vi "Configure Channel (mA Scale).vi"(0 "VISA resource name":refnum<visa-resource-name>, 1 "Scaling":T2={"Floating Point Position (2)"=2, "Lower Scaling (0.00)"=0.0, "Upper Scaling (100.00)"=100.0, "Unit Character (\"\")"=""} {"Upper Scaling (100.00)" format="%_6g"; "Lower Scaling (0.00)" format="%_6g"; "Floating Point Position (2)" min=0 max=5 step=1}, 5 "Channel (0001)":string="0001", 7 "Enable Channel (True)":bool=TRUE, 9 "Range And Span":T1={"mA Range (0 : 0-20mA)"=0, "Enable Span (False)"=FALSE, "Lower Span (0.000)"=0.0, "Upper Span (20.000)"=20.0, "Bias (0)"=0.0} {"mA Range (0 : 0-20mA)" items=["0-20mA"]; "Bias (0)" format="%_6g"; "Upper Span (20.000)" step=0.001 format="%.3g"; "Lower Span (0.000)" step=0.001 format="%.3g"}, 11 "error in (no error)":errorcluster) -> (4 "VISA resource name out":refnum<visa-resource-name>, 6 "Channel":string, 15 "error out":errorcluster)   [LabVIEW 2020, in "Yokogawa GX Series.lvlib"]
doc: "Sets the input range as voltage.\n\nCommand: SRangeAI"
uses:
  <instrlib>/Yokogawa GX Series/Yokogawa GX Series.lvlib
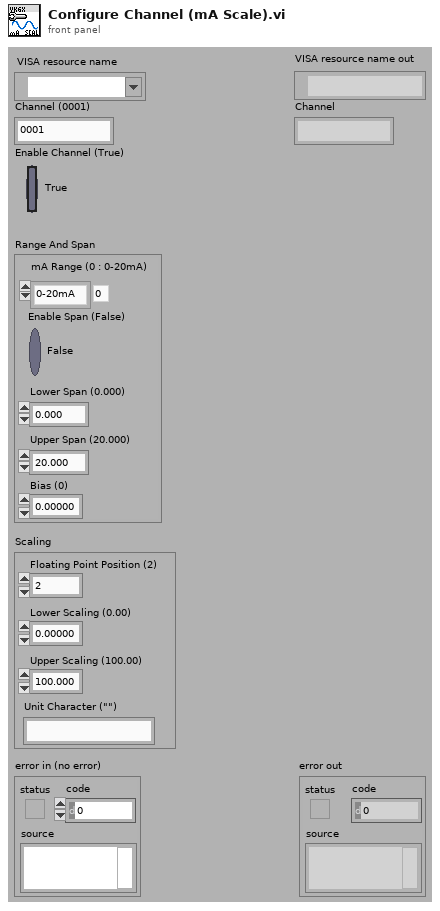
[diagram p1: front panel]
types:
  T1 = cluster{"mA Range (0 : 0-20mA)":i32, "Enable Span (False)":bool, "Lower Span (0.000)":dbl, "Upper Span (20.000)":dbl, "Bias (0)":dbl}
  T2 = cluster{"Floating Point Position (2)":i32, "Lower Scaling (0.00)":dbl, "Upper Scaling (100.00)":dbl, "Unit Character (\"\")":string}
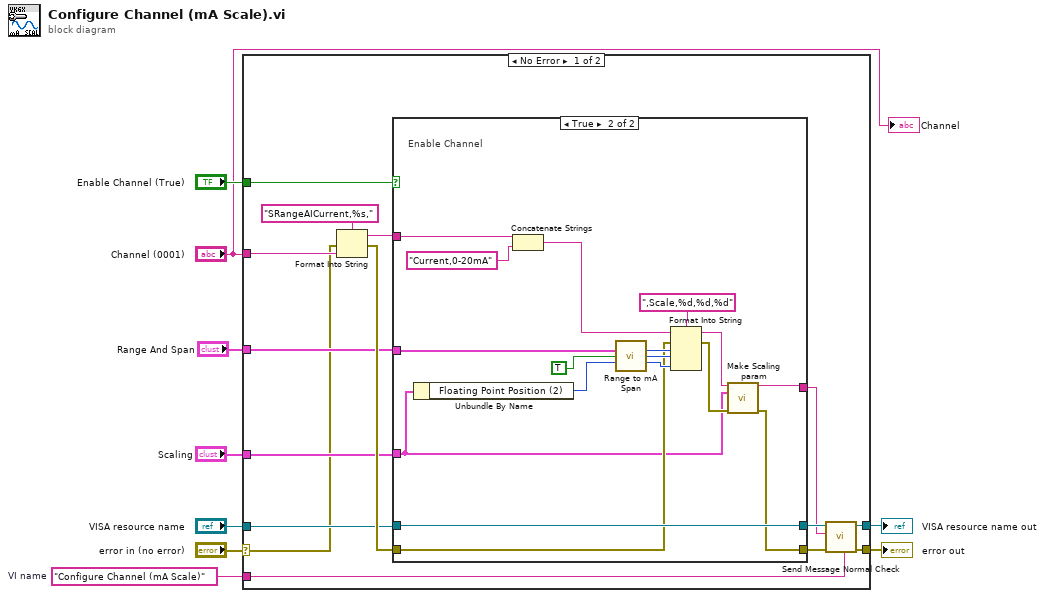
[diagram p0: block diagram]
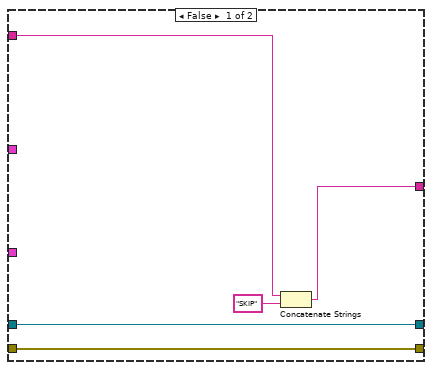
[diagram p2: hidden frame]
diagram:
  w5 = "Configure Channel (mA Scale)"  # VI name
  n1 = case shown="No Error" "error in (no error)" {
    selector: "error in (no error)" -> [w10 w47]
    tunnel: "VISA resource name" -> [w21 w48]
    tunnel: "Scaling" -> [w20 _]
    tunnel: [w17 w48] -> w7
    tunnel: [w16 w47] -> w6
    tunnel: w5 -> [w14 _]
    tunnel: "Range And Span" -> [w13 _]
    tunnel: "Enable Channel (True)" -> [w12 _]
    tunnel: "Channel (0001)" -> [w11 _]
    frame No Error {
      n2 = Format Into String(format string="SRangeAICurrent,%s,", error in=w10, w11) -> (resulting string=w22:string, error out=w23:errorcluster)  [unwired: 1 in]
      n3 = case shown="True" w12 {
        tunnel: w23 -> [w26 w40]
        tunnel: [w26 w37] -> w18
        tunnel: w22 -> [w28 w45]
        tunnel: [w29 w35] -> w15
        tunnel: w21 -> [w25 w41]
        tunnel: [w25 w41] -> w19
        tunnel: w20 -> [_ w33]
        tunnel: w13 -> [_ w31]
        frame False {
          n4 = Concatenate Strings(w28, "SKIP") -> (w29:string)
        }
        frame True {
          # "Enable Channel"
          n5 = Unbundle By Name(w33) -> ("Floating Point Position (2)"=w36:i32)
          n6 = Concatenate Strings(w45, "Current,0-20mA") -> (w30:string)
          n7 = call <instrlib>:"Range to mA Span.vi"("Span"=w31, "Scaling? (False)"=TRUE, "Floating Point Position (2)"=w36) -> ("Lower Span"=w44:i32, "Upper Span"=w43:i32, "Bias"=w42:i32)  [unwired: 10 in]
          n8 = Format Into String(format string=",Scale,%d,%d,%d", initial string=w30, error in=w40, w44, w43, w42) -> (resulting string=w34:string, error out=w38:errorcluster)
          n9 = call <instrlib>:"Make Scaling param.vi"("String (\"\")"=w34, "Scaling"=w33, "error in (no error)"=w38) -> ("String After"=w35:string, "error out"=w37:errorcluster)  [unwired: 11 in]
        }
      }
      n10 = call <instrlib>:"Send Message Normal Check.vi"("Source (\"\")"=w14, "error in (no error)"=w18, "Send Message (\"\")"=w15, "VISA resource name"=w19) -> ("error out"=w16:errorcluster, "VISA resource name out"=w17:refnum<visa-resource-name>)  [unwired: 2 in, 4 out]
    }
    frame Error {
    }
  }
  "error out" <- w6
  "VISA resource name out" <- w7
  "Channel" <- "Channel (0001)"
